vi "Log File Root Properties.vi"(8 "error in":errorcluster, 9 "Author":string, 10 "Description":string, 11 "Title":string) -> (0 "error out":errorcluster, 1 "Author":string, 2 "Description":string, 3 "Title":string)   [LabVIEW 2014]
doc: "<B>Copyrights</B>: (c) MHWirth 2015. All rights reserved.\n\nThis subVI updates the settings for data logging."
panel:
  in  "update":bool
  # "Logging Preference"
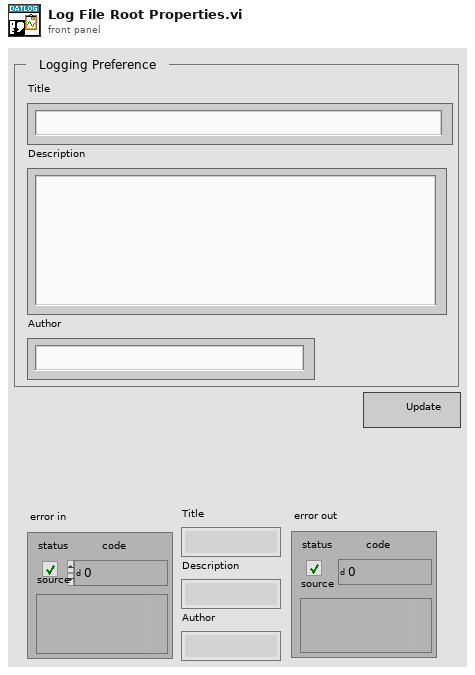
[diagram p1: front panel]
types:
  T1 = typedef "eventvkey.ctl" = enum16{"ASCII", "Enter", "Return", "Shift", "Ctrl", "Alt", "Cmd", "Opt", "Caps", "NumLock", "Clear", "Break", "Up", "Down", "Left", "Right", "Insert", "Delete", "Home", "End", "PageUp", "PageDown", "Escape", "Help", "Pause", "ScrollLock", "F1", "F2", "F3", "F4", "F5", "F6", "F7", "F8", "F9", "F10", "F11", "F12", "F13", "F14", "F15", "F16", "F17", "F18", "F19", "F20", "F21", "F22", "F23", "F24", "Play", "VolumeUp", "VolumeDown", "Mute", "Two Byte Char"}
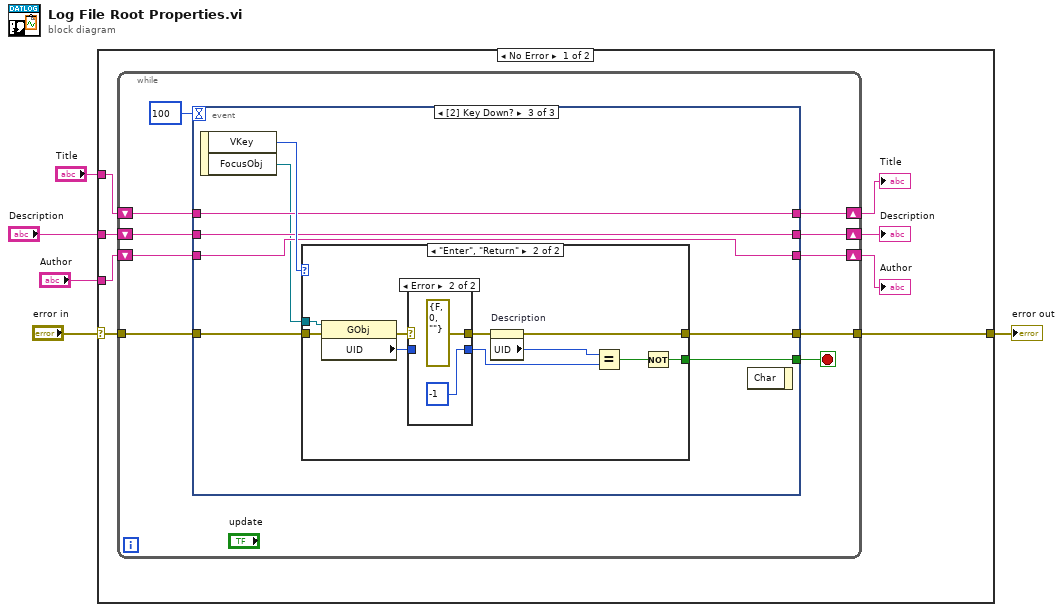
[diagram p0: block diagram]
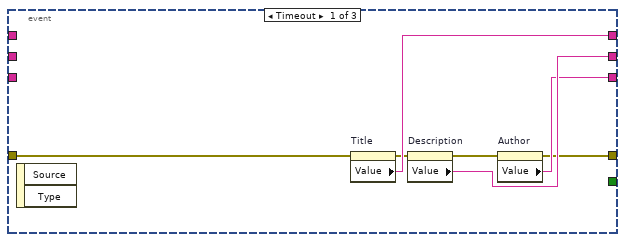
[diagram p2: hidden frame]
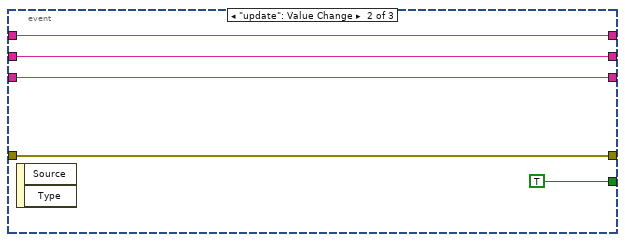
[diagram p3: hidden frame]
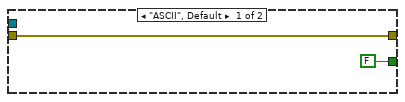
[diagram p4: hidden frame]
diagram:
  n1 = case shown="No Error" "error in" {
    selector: "error in" -> [w13 w60]
    tunnel: [w12 w60] -> w5
    tunnel: "Title" -> [w11 _]
    tunnel: "Description" -> [w9 _]
    tunnel: "Author" -> [w8 _]
    frame No Error {
      n2 = while {
        shift-right: [w20] -> w10
        shift-left: w11 -> [w23]
        shift-right: [w19] -> w6
        shift-left: w8 -> [w22]
        tunnel: w13 -> [w17]
        tunnel: [w16] -> w12
        shift-right: [w14] -> w7
        shift-left: w9 -> [w15]
        stop <- w18 stop-if-true
        n3 = event shown="[2] Key Down?" {
          selector: _ -> [_ _ _]
          dyn-events: _ -> [_ _ _]
          timeout: u32 100 ("milliseconds to wait") -> [_ _ _]
          tunnel: w23 -> [_ w34 w41]
          tunnel: w22 -> [_ w33 w39]
          tunnel: [w30 w34 w41] -> w20
          tunnel: [w25 w33 w39] -> w19
          tunnel: [_ TRUE w42] -> w18
          tunnel: w17 -> [w29 w32 w38]
          tunnel: [w24 w32 w37] -> w16
          tunnel: w15 -> [_ w31 w40]
          tunnel: [w26 w31 w40] -> w14
          event Timeout {
            n4 = event-data() -> ()  [unwired: 1 in, 2 out]
            n5 = property on="Title" class="Str"(error in=w29) -> (error out=w28:errorcluster, "Value"=w30:string)  [unwired: 1 in, 1 out]
            n6 = property on="Description" class="Str"(error in=w28) -> (error out=w27:errorcluster, "Value"=w26:string)  [unwired: 1 in, 1 out]
            n7 = property on="Author" class="Str"(error in=w27) -> (error out=w24:errorcluster, "Value"=w25:string)  [unwired: 1 in, 1 out]
          }
          event "update": Value Change {
            n8 = event-data() -> ()  [unwired: 1 in, 2 out]
          }
          event Key Down? {
            n9 = event-data() -> ("VKey"=w43:T1, "FocusObj"=w36:refnum<vi>)  [unwired: 1 in]
            n10 = case shown="\"Enter\", \"Return\"" w43 {
              tunnel: [FALSE w54] -> w42
              tunnel: w38 -> [w44 w52]
              tunnel: [w44 w55] -> w37
              tunnel: w36 -> [_ w51]
              frame "ASCII", Default {
              }
              frame "Enter", "Return" {
                n11 = property class="GObj"(reference=w51, error in=w52) -> (error out=w49:errorcluster, "UID"=w48:i32)  [unwired: 1 out]
                n12 = case shown="Error" w49 {
                  selector: w49 -> [w56 _]
                  tunnel: w48 -> [w57 _]
                  tunnel: [w57 -1 ("UID")] -> w47
                  tunnel: [w56 errorcluster {"status"=FALSE, "code"=0, "source"=""} ("error IO")] -> w46
                  frame No Error {
                  }
                  frame Error {
                  }
                }
                n13 = property on="Description" class="Str"(error in=w46) -> (error out=w55:errorcluster, "UID"=w50:i32)  [unwired: 1 in, 1 out]
                n14 = Equal?(x=w50, y=w47) -> (x = y?=w53:bool)
                n15 = Not(x=w53) -> (.not. x?=w54:bool)
              }
            }
            n16 = event-data() -> ()  [unwired: 2 in, 1 out]
          }
        }
      }
      "Title" <- w10
      "Description" <- w7
      "Author" <- w6
    }
    frame Error {
    }
  }
  "error out" <- w5
